vi "Configure Timebase.vi"   [LabVIEW 2010, in "Agilent 2000 3000 X-Series.lvlib"]
doc: "Configures timebase settings."
uses:
  <instrlib>/Agilent 2000 3000 X-Series/Agilent 2000 3000 X-Series.lvlib
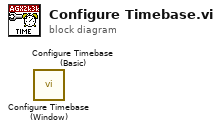
[diagram p0: block diagram]
diagram:
  n1 = call <instrlib>:"Configure Timebase (Window).vi"() -> ()  [unwired: 14 in, 2 out]
  n2 = call <instrlib>:"Configure Timebase (Basic).vi"() -> ()  [unwired: 14 in, 2 out]
